vi "Get CANPorts.vi"(8 "error in (no error)":errorcluster, 11 "Device Item Ref in":T1 format="%.0x") -> (0 "error out":errorcluster, 2 "CAN Ports":string[](array[string]), 3 "Device Item Ref out":T1 format="%.0x")   [LabVIEW 2018, in "CAN Gateway System Explorer.lvlib"]
uses:
  CAN Gateway System Explorer.lvlib
  <vilib>/NI Veristand/Custom Device API/Custom Device Item Ref.ctl
  <vilib>/nisyscfg/Close (System).vi
  <vilib>/regexp/Match Regular Expression.xnode
  <vilib>/nisyscfg/nisyscfg.lvlib
  <resource>/objmgr/nicontrollersysapi.rc
  <vilib>/NI Veristand/Custom Device API/Custom Device API.lvlib
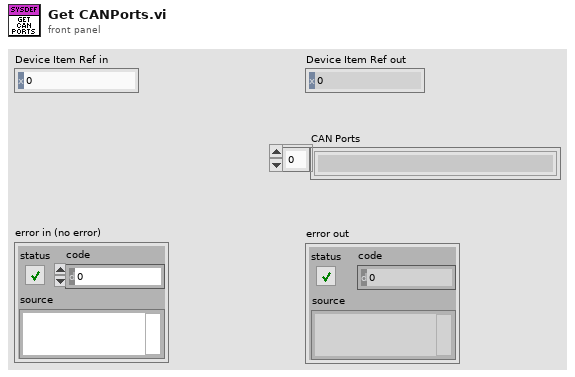
[diagram p1: front panel]
types:
  T1 = typedef "Custom Device API.lvlib/Custom Device Item Ref.ctl" = u64
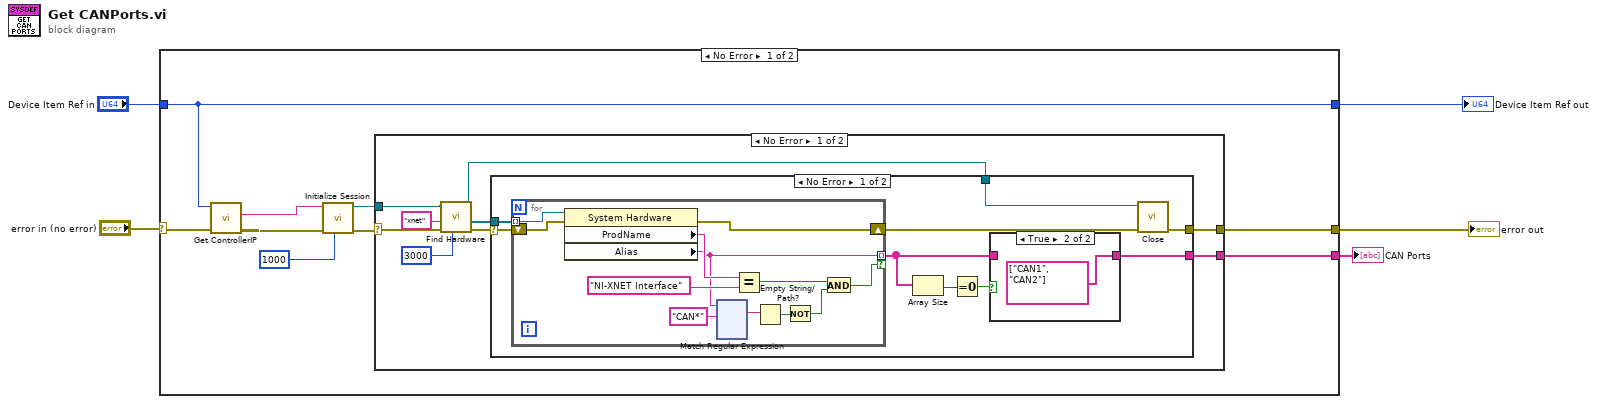
[diagram p0: block diagram]
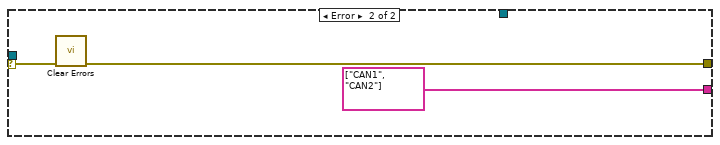
[diagram p3: hidden frame]
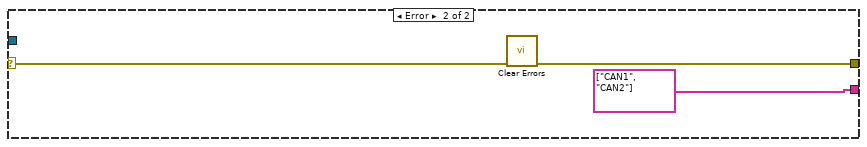
[diagram p4: hidden frame]
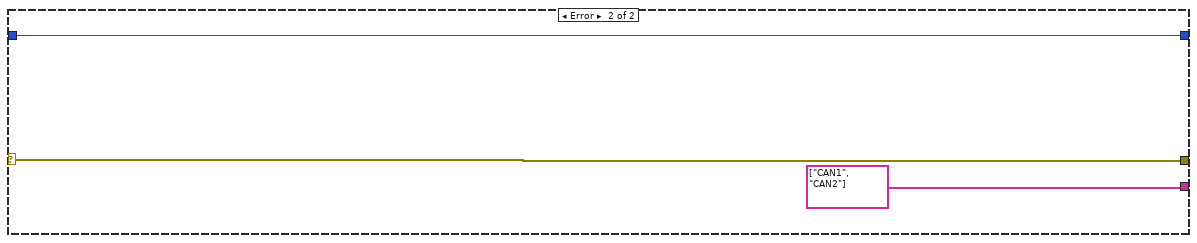
[diagram p5: hidden frame]
diagram:
  n1 = case shown="No Error" "error in (no error)" {
    selector: "error in (no error)" -> [w12 w169]
    tunnel: "Device Item Ref in" -> [w11 w168]
    tunnel: [w11 w168] -> w3
    tunnel: [w13 w169] -> w2
    tunnel: [w6 string[] ["CAN1", "CAN2"]] -> w1
    frame No Error {
      n2 = call "Get ControllerIP.vi"("error in (no error)"=w12, "Device Item Ref in"=w11) -> ("error out"=w10:errorcluster, "element"=w9:string)  [unwired: 7 in, 1 out]
      n3 = call <vilib>:"Initialize Session.vi"("Connect Timeout (4000 ms)"=u32 1000, "error in (no error)"=w10, "Target (localhost)"=w9) -> ("error out"=w7:errorcluster, "Session out"=w14:refnum<k21>)  [unwired: 7 in]
      n4 = case shown="No Error" w7 {
        selector: w7 -> [w17 w166]
        tunnel: w14 -> [w23 _]
        tunnel: [w18 w165] -> w13
        tunnel: [w15 string[] ["CAN1", "CAN2"]] -> w6
        frame No Error {
          n5 = call <vilib>:"Find Hardware.vi"("Remote Timeout (300,000 ms)"=u32 3000, "error in (no error)"=w17, "Experts"="xnet", "Session in"=w23) -> ("error out"=w22:errorcluster, "Resources out"=w21:refnum<k20>[], "Session out"=w19:refnum<k21>)  [unwired: 4 in, 1 out]
          n6 = case shown="No Error" w22 {
            selector: w22 -> [w31 w163]
            tunnel: w21 -> [w30 _]
            tunnel: w19 -> [w29 _]
            tunnel: [w28 w162] -> w18
            tunnel: [w25 string[] ["CAN1", "CAN2"]] -> w15
            frame No Error {
              n7 = for {
                shift-right: [w44] -> w32
                shift-left: w31 -> [w46]
                tunnel: w30 -> [w45] mode=indexing
                tunnel: [w40] -> w24 mode=indexing if=w35
                n8 = property class="System Hardware"(reference=w45, error in=w46) -> (error out=w44:errorcluster, "ProdName"=w43:string, "Alias"=w40:string)  [unwired: 1 out]
                n9 = xnode "Match Regular Expression"("input string"=w40, "regular expression"="CAN*") -> ("whole match"=w39:string)  [unwired: 4 in, 4 out]
                n10 = Equal?(x=w43, y="NI-XNET Interface") -> (x = y?=w37:bool)
                n11 = Empty String/Path?(string/path=w39) -> (empty?=w38:bool)
                n12 = Not(x=w38) -> (.not. x?=w36:bool)
                n13 = And(x=w37, y=w36) -> (x .and. y?=w35:bool)
              }
              n14 = Array Size(array=w24) -> (size(s)=w27:i32)
              n15 = Equal To 0?(x=w27) -> (x = 0?=w26:bool)
              n16 = case shown="True" w26 {
                tunnel: w24 -> [w33 _]
                tunnel: [w33 string[] ["CAN1", "CAN2"]] -> w25
                frame False {
                }
                frame True {
                }
              }
              n17 = call-poly <vilib>:"Close.vi"("error in (no error)"=w32, "Session in"=w29) -> ("error out"=w28:errorcluster)  [unwired: 9 in]
            }
            frame Error {
              n18 = call <vilib>:"Clear Errors.vi"("error in (no error)"=w163) -> ("error out"=w162:errorcluster)  [unwired: 5 in, 1 out]
            }
          }
        }
        frame Error {
          n19 = call <vilib>:"Clear Errors.vi"("error in (no error)"=w166) -> ("error out"=w165:errorcluster)  [unwired: 5 in, 1 out]
        }
      }
    }
    frame Error {
    }
  }
  "error out" <- w2
  "Device Item Ref out" <- w3
  "CAN Ports" <- w1
